vi "Lab_Temp_PID.vi"(1 "Valve Pos":dbl format="%.2f", 2 "Previous Control Sum":dbl format="%.2f", 3 "Present Value":dbl=15.0 format="%.2f", 4 "Setpoint":dbl=15.0 format="%.2f") -> (0 "Dem Output":dbl format="%.2f")   [LabVIEW 2012]
uses:
  <vilib>/Analysis/NI_AALPro.lvlib
panel:
  in  "O/P deadband":dbl=0.5 format="%.2f"
  in  "Kp Deadband":dbl format="%.2f"
  in  "Derivative History":i32=20
  out "deadbanded error":dbl format="%.2f"
  in  "P":bool=TRUE
  in  "D":bool=TRUE
  in  "I":bool=TRUE
  out "Waveform Chart":T1(graph)
  in  "Manual Demand":dbl min=-100.0 max=100.0 format="%.2f"
  in  "Manual Override":bool
  out "Control Sum":dbl format="%.2f"
  out "Derivative Term":dbl format="%.2f"
  out "Integral Term":dbl format="%.2f"
  out "error differential":dbl format="%.5f"
  out "Proportional Term":dbl format="%.2f"
  in  "Kd":dbl=50.0 format="%.2f"
  in  "Ki":dbl=0.025 format="%.3f"
  in  "Kp":dbl=30.0 format="%.2f"
  out "error":dbl format="%.2f"
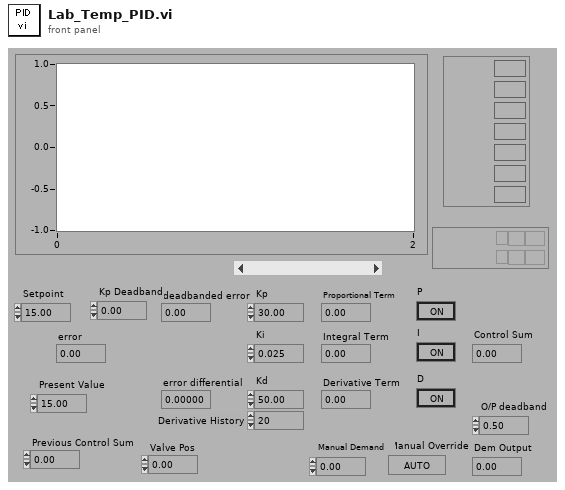
[diagram p1: front panel]
types:
  T1 = cluster{"Setpoint":dbl, "Present Value":dbl, "Proportional Term":dbl, "Integral Term":dbl, "Derivative Term":dbl, "Control Sum":dbl, "Dem Output":dbl}
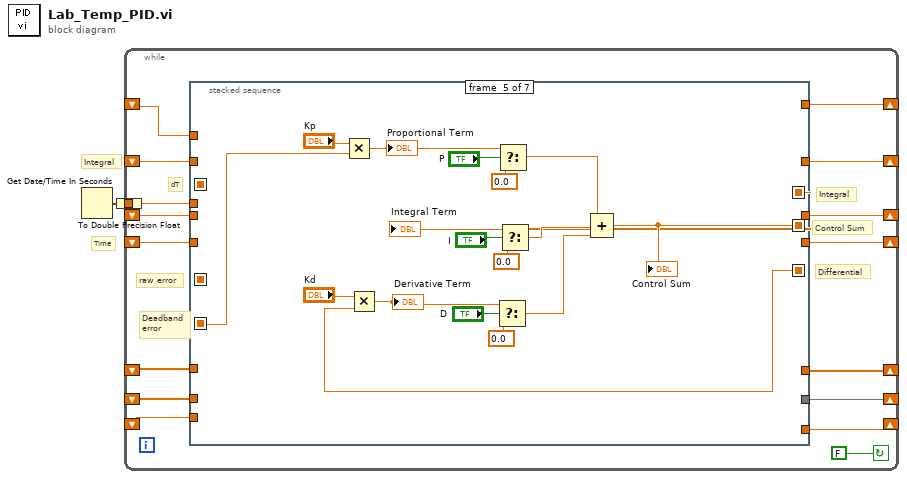
[diagram p0: block diagram]
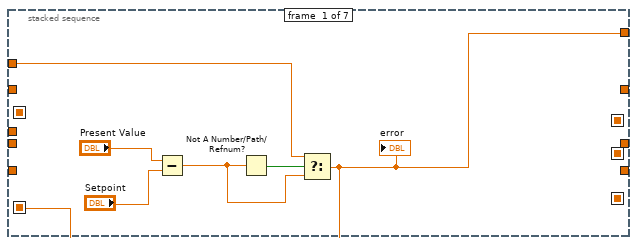
[diagram p2: hidden frame]
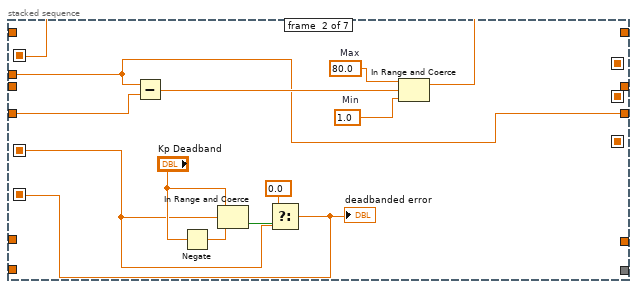
[diagram p3: hidden frame]
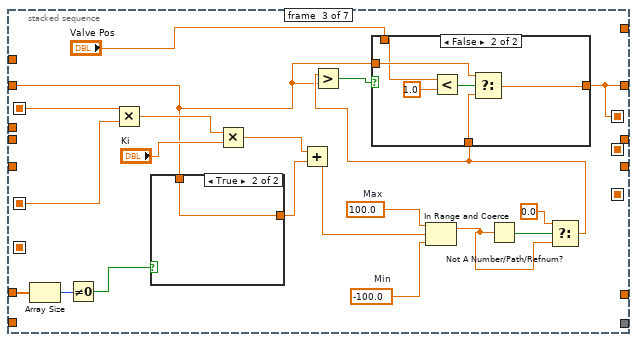
[diagram p4: hidden frame]
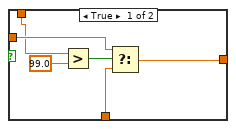
[diagram p5: hidden frame]
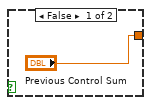
[diagram p6: hidden frame]
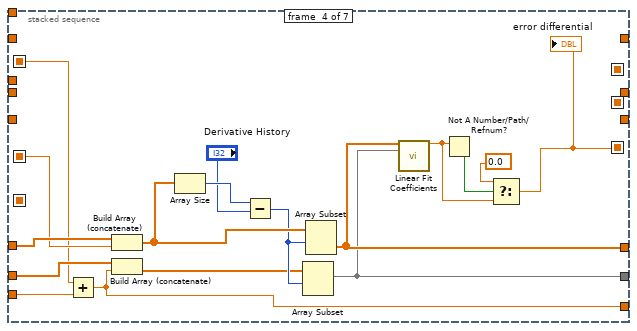
[diagram p7: hidden frame]
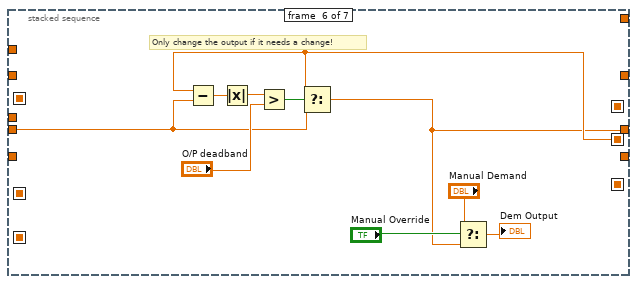
[diagram p8: hidden frame]
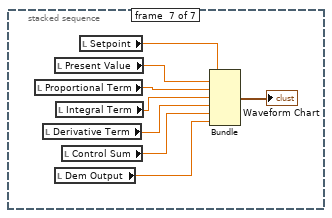
[diagram p9: hidden frame]
diagram:
  # "Integral"
  # "Time"
  n1 = Get Date/Time In Seconds() -> (seconds since 1Jan1904=w1:timestamp)
  n2 = To Double Precision Float(number=w1) -> (double precision float=w2:dbl)
  n3 = while {
    shift-left: _ -> [w5]
    shift-right: [w4] -> _
    shift-left: _ -> [w7]
    shift-right: [w6] -> _
    shift-left: _ -> [w9]
    shift-right: [w8] -> _
    tunnel: w2 -> [w14]
    shift-left: _ -> [w11]
    shift-right: [w10] -> _
    shift-left: _ -> [w13]
    shift-right: [w12] -> _
    shift-left: _ -> [w15]
    shift-right: [w16] -> _
    shift-left: _ -> [w18]
    shift-right: [w17] -> _
    stop <- FALSE continue-if-true
    # "Control Sum"
    # "raw error"
    # "Differential"
    # "Integral"
    # "Deadband\nerror"
    # "dT"
    n4 = stacked-sequence {
      seq-local: [_ w25 _ _ _ _ _] -> [_ _ w56 w73 _ _ _]
      seq-local: [_ w34 _ _ _ _ _] -> [_ _ _ _ w90 _ _]
      seq-local: [_ _ _ w78 _ _ _] -> [_ _ _ _ w89 _ _]
      seq-local: [_ _ w37 _ _ _ _] -> [_ _ _ _ w88 _ _]
      seq-local: [w20 _ _ _ _ _ _] -> [_ w26 w54 w79 _ _ _]
      seq-local: [_ _ _ _ w93 _ _] -> [_ _ _ _ _ w108 _]
      tunnel: w18 -> [_ w31 _ _ _ _ _]
      tunnel: [_ w29 _ _ _ _ _] -> w17
      tunnel: [_ _ w37 _ _ _ _] -> w16
      tunnel: w15 -> [_ _ w39 _ _ _ _]
      tunnel: w14 -> [_ w29 _ _ _ _ _]
      tunnel: w13 -> [_ _ w53 w87 _ _ _]
      tunnel: [_ _ _ w80 _ _ _] -> w12
      tunnel: w11 -> [_ _ _ w86 _ _ _]
      tunnel: [_ _ _ w77 _ _ _] -> w10
      tunnel: w9 -> [_ _ _ _ _ w106 _]
      tunnel: [_ _ _ _ _ w105 _] -> w8
      tunnel: w7 -> [_ _ _ w72 _ _ _]
      tunnel: [_ _ _ w71 _ _ _] -> w6
      tunnel: w5 -> [w21 _ _ _ _ _ _]
      tunnel: [w20 _ _ _ _ _ _] -> w4
      frame #0 {
        n5 = Subtract(x="Present Value", y="Setpoint") -> (x-y=w19:dbl)
        n6 = Not A Number/Path/Refnum?(number/path/refnum=w19) -> (NaN/Path/Refnum?=w22:bool)
        n7 = Select(t=w21, s=w22, f=w19) -> (s? t:f=w20:dbl)
        "error" <- w20
      }
      frame #1 {
        w32 = 1.0  # Min
        w33 = 80.0  # Max
        n8 = Subtract(x=w29, y=w31) -> (x-y=w30:dbl)
        n9 = Negate(x="Kp Deadband") -> (-x=w28:dbl)
        n10 = In Range and Coerce(upper limit="Kp Deadband", x=w26, lower limit=w28) -> (In Range?=w35:bool)  [unwired: 1 out]
        n11 = Select(t=0.0, s=w35, f=w26) -> (s? t:f=w34:dbl)
        "deadbanded error" <- w34
        n12 = In Range and Coerce(upper limit=w33, x=w30, lower limit=w32) -> (coerced(x)=w25:dbl)  [unwired: 1 out]
      }
      frame #2 {
        w42 = -100.0  # Min
        w43 = 100.0  # Max
        n13 = Array Size(array=w53) -> (size(s)=w52:i32)
        n14 = Not Equal To 0?(x=w52) -> (x != 0?=w51:bool)
        n15 = Multiply(x=w56, y=w54) -> (x*y=w46:dbl)
        n16 = case shown="True" w51 {
          tunnel: ["Previous Control Sum" w70] -> w50
          tunnel: w39 -> [_ w70]
          frame False {
          }
          frame True {
          }
        }
        n17 = Multiply(x=w46, y="Ki") -> (x*y=w44:dbl)
        n18 = Add(x=w44, y=w50) -> (x+y=w55:dbl)
        n19 = In Range and Coerce(upper limit=w43, x=w55, lower limit=w42) -> (coerced(x)=w48:dbl)  [unwired: 1 out]
        n20 = Not A Number/Path/Refnum?(number/path/refnum=w48) -> (NaN/Path/Refnum?=w49:bool)
        n21 = Select(t=0.0, s=w49, f=w48) -> (s? t:f=w40:dbl)
        n22 = Greater?(x=w40, y=w39) -> (0:w41:bool)
        n23 = case shown="False" w41 {
          tunnel: w40 -> [w62 w68]
          tunnel: w39 -> [w61 w67]
          tunnel: [w60 w66] -> w37
          tunnel: "Valve Pos" -> [w58 w64]
          frame True {
            n24 = Greater?(x=w58, y=99.0) -> (0:w57:bool)
            n25 = Select(t=w61, s=w57, f=w62) -> (s? t:f=w60:dbl)
          }
          frame False {
            n26 = Less?(x=w64, y=1.0) -> (x < y?=w63:bool)
            n27 = Select(t=w67, s=w63, f=w68) -> (s? t:f=w66:dbl)
          }
        }
      }
      frame #3 {
        n28 = Add(x=w73, y=w72) -> (x+y=w71:dbl)
        n29 = Build Array (concatenate)(w87, w79) -> (w83:dbl[])
        n30 = Build Array (concatenate)(w86, w71) -> (w81:dbl[])
        n31 = Array Size(array=w83) -> (size(s)=w85:i32)
        n32 = Subtract(x=w85, y="Derivative History") -> (x-y=w82:i32)
        n33 = Array Subset(array=w81, index=w82) -> (w77:dbl[])  [unwired: 1 in]
        n34 = Array Subset(array=w83, index=w82) -> (w80:dbl[])  [unwired: 1 in]
        n35 = call <vilib>:"Linear Fit Coefficients.vi"("Y"=w80, "X"=w77) -> ("slope"=w74:dbl)  [unwired: 3 in, 10 out]
        n36 = Not A Number/Path/Refnum?(number/path/refnum=w74) -> (NaN/Path/Refnum?=w76:bool)
        n37 = Select(t=0.0 ("f"), s=w76, f=w74) -> (s? t:f=w78:dbl)
        "error differential" <- w78
      }
      frame #4 {
        n38 = Multiply(x="Kp", y=w90) -> (x*y=w102:dbl)
        "Proportional Term" <- w102
        n39 = Multiply(x="Kd", y=w89) -> (x*y=w94:dbl)
        "Derivative Term" <- w94
        n40 = Select(t=w94, s="D", f=0.0) -> (s? t:f=w96:dbl)
        n41 = Select(t=w102, s="P", f=0.0) -> (s? t:f=w103:dbl)
        n42 = Select(t=w88, s="I", f=0.0) -> (s? t:f=w95:dbl)
        n43 = Compound Arithmetic op=ADD(w103, w95, w96) -> (w93:dbl)
        "Control Sum" <- w93
        "Integral Term" <- w88
      }
      frame #5 {
        # "Only change the output if it needs a change!"
        n44 = Subtract(x=w108, y=w106) -> (x-y=w111:dbl)
        n45 = Absolute Value(x=w111) -> (abs(x)=w110:dbl)
        n46 = Greater?(x=w110, y="O/P deadband") -> (0:w109:bool)
        n47 = Select(t=w108, s=w109, f=w106) -> (s? t:f=w105:dbl)
        n48 = Select(t="Manual Demand", s="Manual Override", f=w105) -> (s? t:f=→"Dem Output":dbl)
      }
      frame #6 {
        n49 = local read "Proportional Term"() -> (w118:dbl)
        n50 = local read "Derivative Term"() -> (w120:dbl)
        n51 = local read "Present Value"() -> (w117:dbl)
        n52 = local read "Dem Output"() -> (w122:dbl)
        n53 = local read "Integral Term"() -> (w119:dbl)
        n54 = local read "Control Sum"() -> (w121:dbl)
        n55 = local read "Setpoint"() -> (w116:dbl)
        n56 = Bundle("Setpoint"=w116, "Present Value"=w117, "Proportional Term"=w118, "Integral Term"=w119, "Derivative Term"=w120, "Control Sum"=w121, "Dem Output"=w122) -> (→"Waveform Chart":T1)  [unwired: 1 out]
      }
    }
  }
